vi "PORT IO Read Byte__ogtk.vi"(4 "error in (no error)":errorcluster, 5 "fast (F)":bool, 6 "type":u8, 7 "address":u16 format="%.0x") -> (0 "error out":errorcluster, 2 "value":u8)   [LabVIEW 2018]
doc: "This function reads in a single byte from the specified IO port. If you set fast to True, and are running under Windows NT/2000/XP/2003 you must have enabled the according IO port with a call to \"PORT IO Enable Range.vi\" to avoid a General Protection Fault error."
uses:
  <userlib>/_OpenG.lib/portio/ogportio.dll
panel:
  # "[OpenG VI Tags] ***Do Not Remove***"
  # "PORT IO Read Byte.vi\n\nReads a byte from the port IO range.\n\nPlease visit http://www.OpenG.org to learn about the\nOpen Source LabVIEW software movement.\n\nNOTICE -- YOU MUST LEAVE THIS NOTICE IN PLACE.  PER THE TERMS OF THE LICENSE BELOW, YOU MAY SUBLICENSE THIS SOFTWARE \nIN ANY WAY THAT DOES NOT CONFLICT WITH THIS LICENSE.\n\n### BSD License (http://www.opensource.org/licenses/bsd-license.php) Begin ###\n\nCopyright (c) 2002-2007, Rolf Kalbermatter <rolf.kalbermatter@citeng.com> \n\nAll rights reserved.\n\nRedistribution and use in source and binary forms, with or without modification, are permitted provided that the following conditions are met:\n\n    * Redistributions of source code must retain the above copyright notice, this list of conditions and the following disclaimer.\n    * Redistributions in binary form must reproduce the above copyright notice, this list of conditions and the following disclaimer in the \n       documentation and/or other materials provided with the distribution.\n    * Neither the name of SciWare, James Kring, Inc., nor the names of its contributors may be used to endorse or promote products derived \n       from this software without specific prior written permission.\n\nTHIS SOFTWARE IS PROVIDED BY THE COPYRIGHT HOLDERS AND CONTRIBUTORS \"AS IS\" AND ANY EXPRESS OR IMPLIED WARRANTIES, \nINCLUDING, BUT NOT LIMITED TO, THE IMPLIED WARRANTIES OF MERCHANTABILITY AND FITNESS FOR A PARTICULAR PURPOSE ARE \nDISCLAIMED. IN NO EVENT SHALL THE COPYRIGHT OWNER OR CONTRIBUTORS BE LIABLE FOR ANY DIRECT, INDIRECT, INCIDENTAL,\n SPECIAL, EXEMPLARY, OR CONSEQUENTIAL DAMAGES (INCLUDING, BUT NOT LIMITED TO, PROCUREMENT OF SUBSTITUTE GOODS OR \nSERVICES; LOSS OF USE, DATA, OR PROFITS; OR BUSINESS INTERRUPTION) HOWEVER CAUSED AND ON ANY THEORY OF LIABILITY, \nWHETHER IN CONTRACT, STRICT LIABILITY, OR TORT (INCLUDING NEGLIGENCE OR OTHERWISE) ARISING IN ANY WAY OUT OF THE USE \nOF THIS SOFTWARE, EVEN IF ADVISED OF THE POSSIBILITY OF SUCH DAMAGE.\n\n### BSD License End ###"
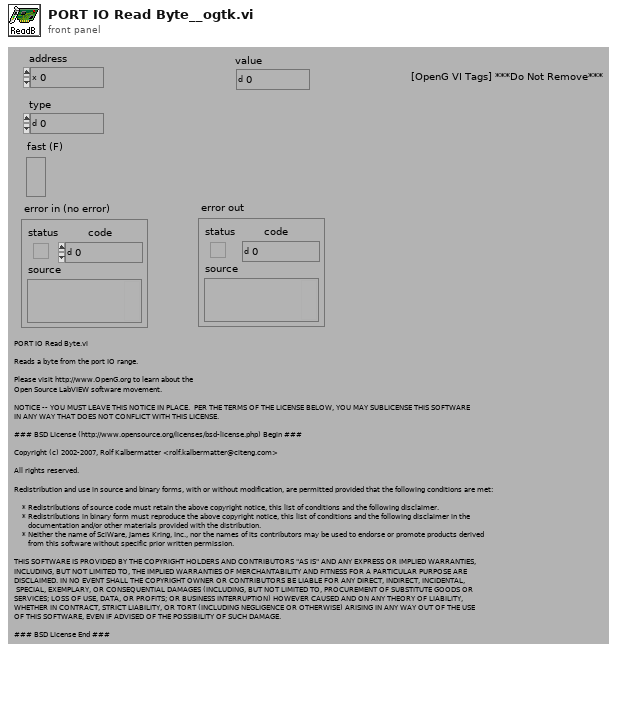
[diagram p1: front panel]
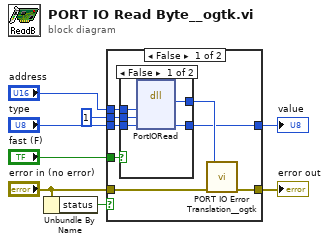
[diagram p0: block diagram]
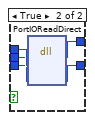
[diagram p2: hidden frame]
diagram:
  n1 = Unbundle By Name("error in (no error)") -> ("status"=w8:bool)
  n2 = case shown="False" w8 {
    tunnel: "error in (no error)" -> [w10 w28]
    tunnel: "address" -> [w15 _]
    tunnel: "type" -> [w14 w27]
    tunnel: [w13 w27] -> w4
    tunnel: u32 1 ("process") -> [w12 _]
    tunnel: "fast (F)" -> [w11 _]
    tunnel: [w9 w28] -> w1
    frame False {
      n3 = case shown="False" w11 {
        tunnel: [w18 w26] -> w16
        tunnel: w15 -> [w19 w25]
        tunnel: w14 -> [w21 w24]
        tunnel: [w17 w23] -> w13
        tunnel: w12 -> [w20 w22]
        frame False {
          n4 = dll-call lib="D:/src/DRVSRC/iosys/ogportio/ogportio.*" fn="PortIORead"("address"=w19, "size"=w20, "type"=w21) -> (w18:u32, "type"=w17:u8)  [unwired: 5 in, 2 out]
        }
        frame True {
          n5 = dll-call lib="D:/Projects/OpenG/opengtoolkit/portIO/source/ogportio.*" fn="PortIOReadDirect"("address"=w25, "size"=w22, "type"=w24) -> (w26:u32, "type"=w23:u8)  [unwired: 5 in, 2 out]
        }
      }
      n6 = call <userlib>:"PORT IO Error Translation__ogtk.vi"("error in (no error)"=w10, "win error"=w16) -> ("error out"=w9:errorcluster)  [unwired: 5 in]
    }
    frame True {
    }
  }
  "error out" <- w1
  "value" <- w4
